vi "LightningPID.vi"(8 "PID Settings":T1, 9 "Reset":bool, 10 "Position":dbl, 11 "Set Point":dbl) -> (3 "Output":dbl)   [LabVIEW 2014]
panel:
  out "dBase":dbl(graph)
  out "iState":dbl(graph)
  out "dBase":dbl
  out "iState":dbl
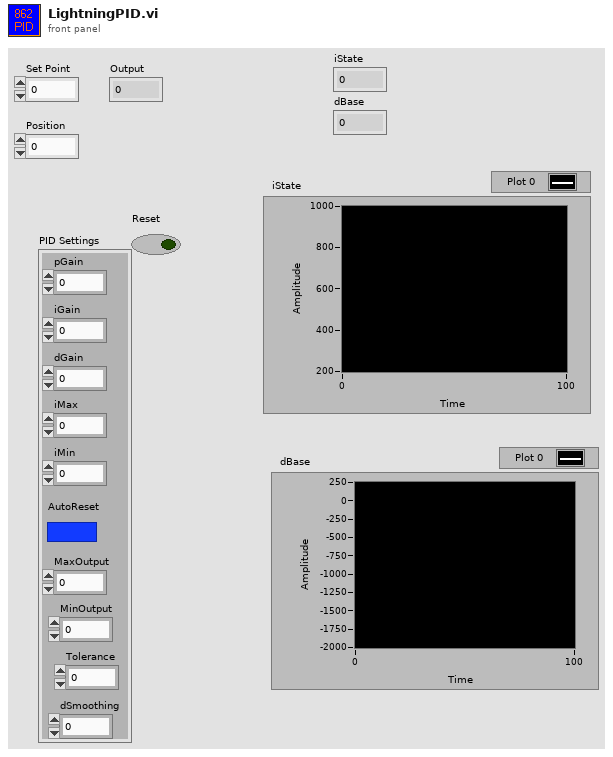
[diagram p1: front panel]
types:
  T1 = cluster{"iMax":dbl, "iMin":dbl, "iGain":dbl, "pGain":dbl, "dGain":dbl, "MaxOutput":dbl, "MinOutput":dbl, "AutoReset":bool, "Tolerance":dbl, "dSmoothing":dbl}
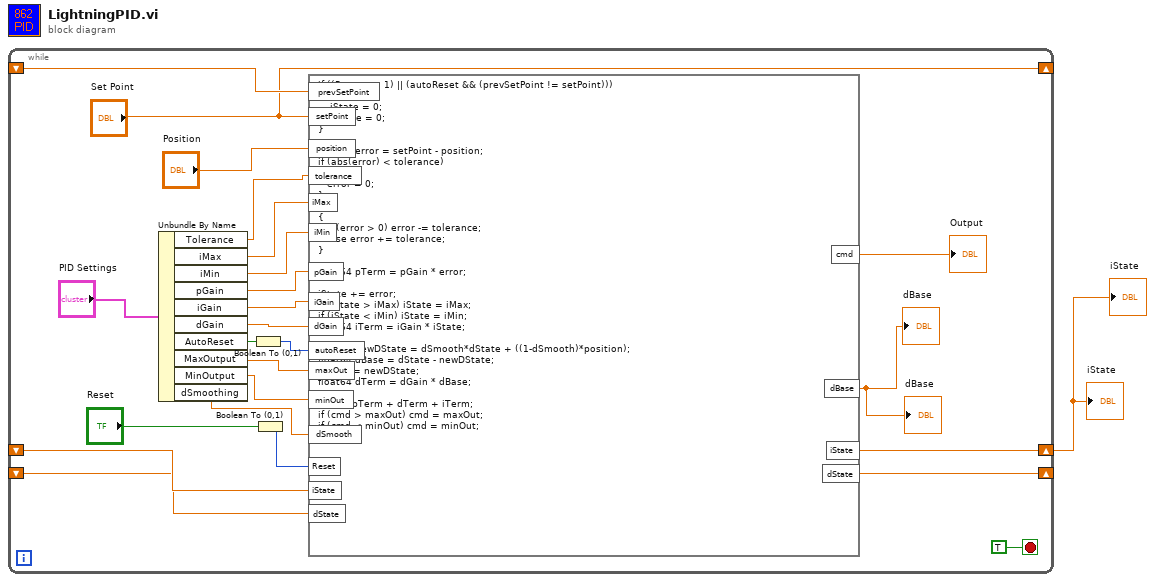
[diagram p0: block diagram]
diagram:
  n1 = while {
    shift-right: [w18] -> w1
    shift-left: _ -> [w16]
    shift-right: [w17] -> _
    shift-left: _ -> [w15]
    shift-right: ["Set Point"] -> _
    shift-left: _ -> [w14]
    stop <- TRUE stop-if-true
    n2 = Unbundle By Name("PID Settings") -> ("Tolerance"=w3:dbl, "iMax"=w23:dbl, "iMin"=w5:dbl, "pGain"=w22:dbl, "iGain"=w21:dbl, "dGain"=w20:dbl, "AutoReset"=w12:bool, "MaxOutput"=w7:dbl, "MinOutput"=w6:dbl, "dSmoothing"=w2:dbl)
    n3 = Boolean To (0,1)(Boolean=w12) -> (0, 1=w13:i16)
    n4 = Boolean To (0,1)(Boolean="Reset") -> (0, 1=w11:i16)
    n5 = formula code="if ((Reset == 1) || (autoReset && (prevSetPoint != setPoint)))\n{\n    iState = 0;\n    dState = 0;\n}\n\nfloat64 error = setPoint - position;\nif (abs(error) < tolerance) \n{\n   error = 0;\n}\nelse\n{\n   if (error > 0) error -= tolerance;\n   else error += tolerance;\n}\n\nfloat64 pTerm = pGain * error;\n\niState += error;\nif (iState > iMax) iState = iMax;\nif (iState < iMin) iState = iMin;\nfloat64 iTerm = iGain * iState;\n\nfloat64 newDState = dSmooth*dState + ((1-dSmooth)*position);\nfloat64 dBase = dState - newDState;\ndState = newDState;\nfloat64 dTerm = dGain * dBase;\n\ncmd = pTerm + dTerm + iTerm;\nif (cmd > maxOut) cmd = maxOut;\nif (cmd < minOut) cmd = minOut;"("position"="Position", "dState"=w15, "iState"=w16, "pGain"=w22, "iGain"=w21, "dGain"=w20, "iMax"=w23, "iMin"=w5, "Reset"=w11, "prevSetPoint"=w14, "autoReset"=w13, "setPoint"="Set Point", "maxOut"=w7, "minOut"=w6, "tolerance"=w3, "dSmooth"=w2) -> ("cmd"=→"Output":dbl, "iState"=w18:dbl, "dState"=w17:dbl, "dBase"=→"dBase" →"dBase":dbl)
  }
  "iState" <- w1
  "iState" <- w1
